vi "AI algorithm(SubVI).vi"(2 "Turn":bool, 3 "XO array":string[][](array[string])) -> (0 "Turn 2":bool, 1 "XO array 2":string[][](array[string]))   [LabVIEW 2020]
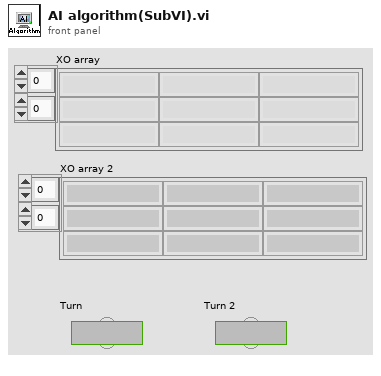
[diagram p1: front panel]
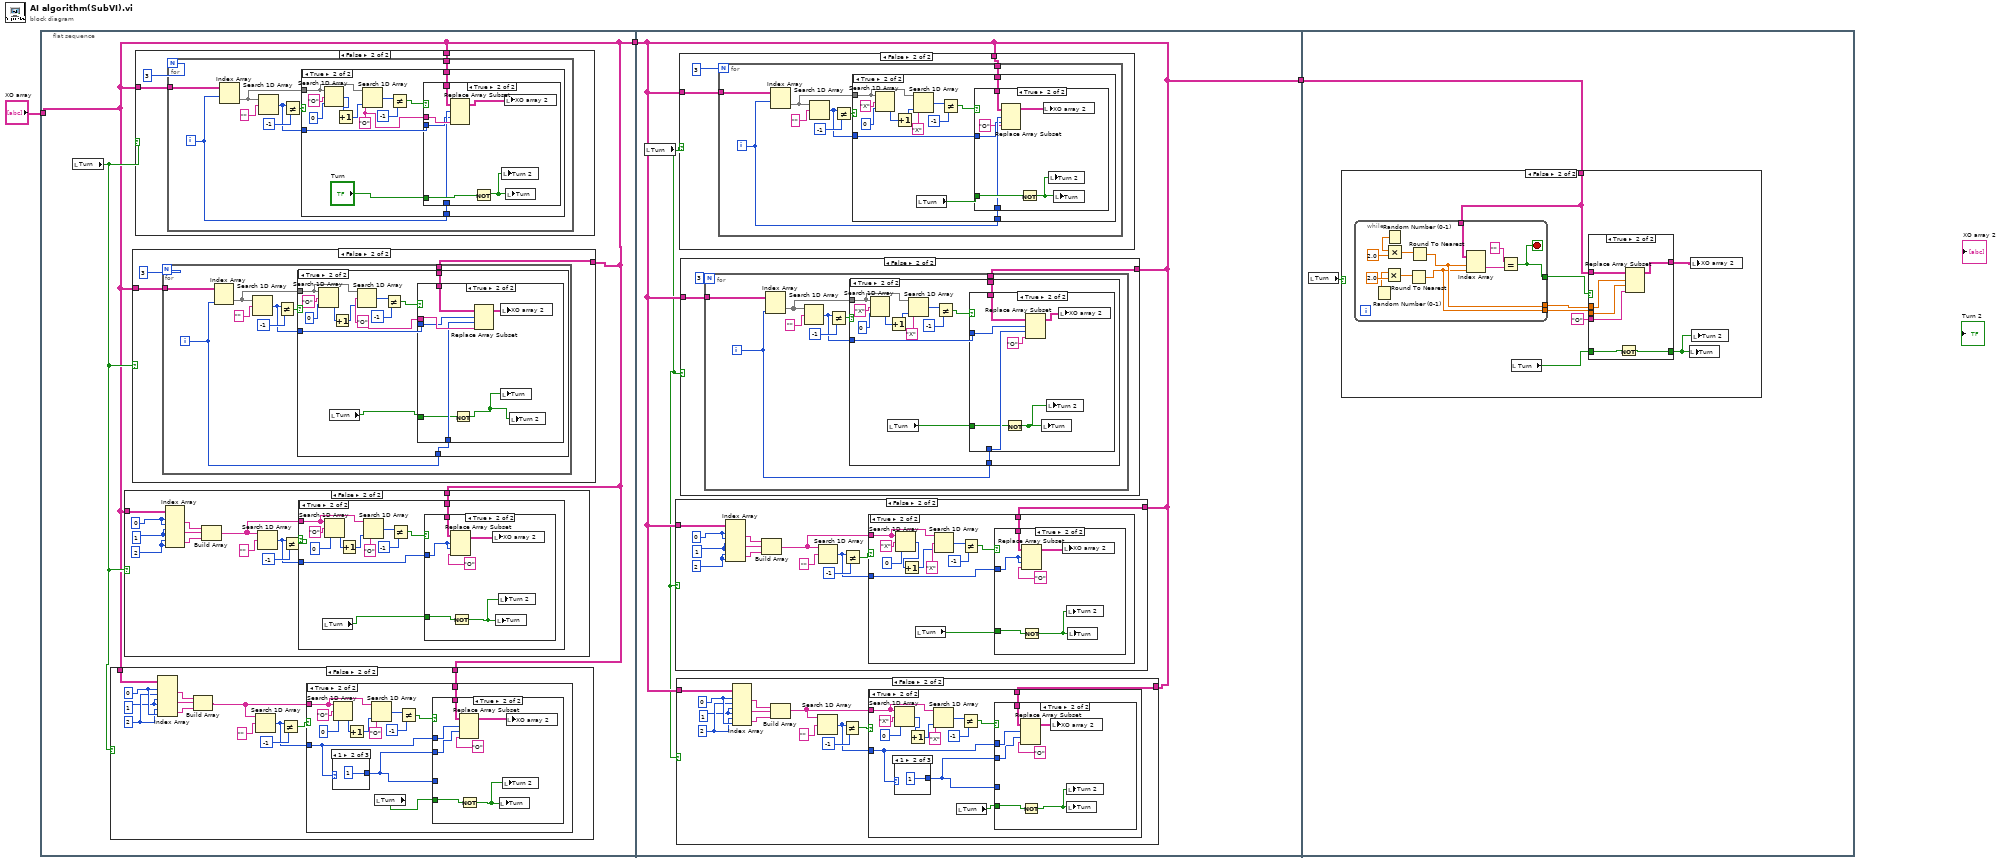
[diagram p0: block diagram]
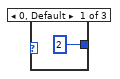
[diagram p4: hidden frame]
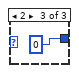
[diagram p5: hidden frame]
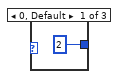
[diagram p18: hidden frame]
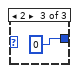
[diagram p19: hidden frame]
diagram:
  n1 = flat-sequence {
    tunnel: "XO array" -> [w4]
    tunnel: [w4] -> w2
    tunnel: w2 -> [w136]
    tunnel: [w136] -> w1
    tunnel: w1 -> [w267]
    frame #0 {
      n2 = local read "Turn"() -> (w5:bool)
      n3 = case shown="False" w5 {
        tunnel: w4 -> [_ w18]
        tunnel: w4 -> [_ w6]
        frame True {
        }
        frame False {
          w13 = 2
          w12 = 1
          w14 = 0
          n4 = Index Array(array=w18, index (row) #1=w14, index (col) #1=w13, index (row) #2=w12, index (col) #2=w12, index (row) #3=w13, index (col) #3=w14) -> (element #1=w17:string, element #2=w16:string, element #3=w15:string)
          n5 = Build Array(w17, w16, w15) -> (w7:string[])
          n6 = Search 1D Array(1D array=w7, element="") -> (index of element=w8:i32)  [unwired: 1 in]
          n7 = Not Equal?(x=w8, y=-1) -> (x != y?=w9:bool)
          n8 = case shown="True" w9 {
            tunnel: w7 -> [_ w30]
            tunnel: w8 -> [_ w24]
            tunnel: w6 -> [_ w25]
            frame False {
            }
            frame True {
              n9 = case shown="1" w24 {
                tunnel: [2 1 0] -> w23
                frame 0, Default {
                }
                frame 1 {
                }
                frame 2 {
                }
              }
              n10 = Search 1D Array(1D array=w30, element="O", start index (0)=0) -> (index of element=w22:i32)
              n11 = Increment(x=w22) -> (x+1=w21:i32)
              n12 = Search 1D Array(1D array=w30, element="O", start index (0)=w21) -> (index of element=w28:i32)
              n13 = local read "Turn"() -> (w20:bool)
              n14 = Not Equal?(x=w28, y=-1) -> (x != y?=w26:bool)
              n15 = case shown="True" w26 {
                tunnel: w24 -> [_ w39]
                tunnel: w25 -> [_ w41]
                tunnel: w20 -> [_ w38]
                tunnel: w23 -> [_ _]
                tunnel: w23 -> [_ w37]
                frame False {
                }
                frame True {
                  n16 = Replace Array Subset(array=w41, new element="O" ("new element/subarray"), index (row)=w39, index (col)=w37) -> (w36:string[][])
                  n17 = Not(x=w38) -> (.not. x?=w35:bool)
                  n18 = local write "Turn"(w35) -> ()
                  n19 = local write "Turn 2"(w35) -> ()
                  n20 = local write "XO array 2"(w36) -> ()
                }
              }
            }
          }
        }
      }
      n21 = case shown="False" w5 {
        tunnel: w4 -> [_ w54]
        tunnel: w4 -> [_ w42]
        frame True {
        }
        frame False {
          w47 = 2
          w48 = 1
          w49 = 0
          n22 = Index Array(array=w54, index (row) #1=w49, index (col) #1=w49, index (row) #2=w48, index (col) #2=w48, index (row) #3=w47, index (col) #3=w47) -> (element #1=w46:string, element #2=w45:string, element #3=w44:string)
          n23 = Build Array(w46, w45, w44) -> (w43:string[])
          n24 = Search 1D Array(1D array=w43, element="") -> (index of element=w50:i32)  [unwired: 1 in]
          n25 = Not Equal?(x=w50, y=-1) -> (x != y?=w51:bool)
          n26 = case shown="True" w51 {
            tunnel: w43 -> [_ w65]
            tunnel: w50 -> [_ w60]
            tunnel: w42 -> [_ w59]
            frame False {
            }
            frame True {
              n27 = local read "Turn"() -> (w56:bool)
              n28 = Search 1D Array(1D array=w65, element="O", start index (0)=0) -> (index of element=w58:i32)
              n29 = Increment(x=w58) -> (x+1=w57:i32)
              n30 = Search 1D Array(1D array=w65, element="O", start index (0)=w57) -> (index of element=w63:i32)
              n31 = Not Equal?(x=w63, y=-1) -> (x != y?=w61:bool)
              n32 = case shown="True" w61 {
                tunnel: w60 -> [_ w70]
                tunnel: w59 -> [_ w72]
                tunnel: w56 -> [_ w69]
                frame False {
                }
                frame True {
                  n33 = Replace Array Subset(array=w72, new element="O" ("new element/subarray"), index (row)=w70, index (col)=w70) -> (w68:string[][])
                  n34 = Not(x=w69) -> (.not. x?=w67:bool)
                  n35 = local write "XO array 2"(w68) -> ()
                  n36 = local write "Turn"(w67) -> ()
                  n37 = local write "Turn 2"(w67) -> ()
                }
              }
            }
          }
        }
      }
      n38 = case shown="False" w5 {
        tunnel: w4 -> [_ w75]
        tunnel: w4 -> [_ w73]
        frame True {
        }
        frame False {
          n39 = for {
            N: 3 -> [_]
            tunnel: w75 -> [w83]
            tunnel: w73 -> [w77]
            i -> [w76]
            n40 = Index Array(array=w83, index (col)=w76) -> (element=w79:string[])  [unwired: 1 in]
            n41 = Search 1D Array(1D array=w79, element="") -> (index of element=w78:i32)  [unwired: 1 in]
            n42 = Not Equal?(x=w78, y=-1) -> (x != y?=w80:bool)
            n43 = case shown="True" w80 {
              tunnel: w79 -> [_ w95]
              tunnel: w78 -> [_ w91]
              tunnel: w77 -> [_ w90]
              tunnel: w76 -> [_ w89]
              frame False {
              }
              frame True {
                w88 = "O" ("element")
                n44 = Search 1D Array(1D array=w95, element="O", start index (0)=0) -> (index of element=w87:i32)
                n45 = local read "Turn"() -> (w85:bool)
                n46 = Increment(x=w87) -> (x+1=w86:i32)
                n47 = Search 1D Array(1D array=w95, element=w88, start index (0)=w86) -> (index of element=w94:i32)
                n48 = Not Equal?(x=w94, y=-1) -> (x != y?=w92:bool)
                n49 = case shown="True" w92 {
                  tunnel: w91 -> [_ w100]
                  tunnel: w90 -> [_ w103]
                  tunnel: w89 -> [_ w101]
                  tunnel: w88 -> [_ w102]
                  tunnel: w85 -> [_ w99]
                  frame False {
                  }
                  frame True {
                    n50 = Not(x=w99) -> (.not. x?=w97:bool)
                    n51 = Replace Array Subset(array=w103, new element=w102, index (row)=w100, index (col)=w101) -> (w98:string[][])
                    n52 = local write "XO array 2"(w98) -> ()
                    n53 = local write "Turn"(w97) -> ()
                    n54 = local write "Turn 2"(w97) -> ()
                  }
                }
              }
            }
          }
        }
      }
      n55 = case shown="False" w5 {
        tunnel: w4 -> [_ w106]
        tunnel: w4 -> [_ w104]
        frame True {
        }
        frame False {
          n56 = for {
            N: 3 -> [_]
            tunnel: w106 -> [w114]
            tunnel: w104 -> [w108]
            i -> [w107]
            n57 = Index Array(array=w114, index (row)=w107) -> (element=w110:string[])  [unwired: 1 in]
            n58 = Search 1D Array(1D array=w110, element="") -> (index of element=w109:i32)  [unwired: 1 in]
            n59 = Not Equal?(x=w109, y=-1) -> (x != y?=w111:bool)
            n60 = case shown="True" w111 {
              tunnel: w110 -> [_ w126]
              tunnel: w109 -> [_ w122]
              tunnel: w108 -> [_ w120]
              tunnel: w107 -> [_ w119]
              frame False {
              }
              frame True {
                w121 = "O" ("element")
                n61 = Search 1D Array(1D array=w126, element="O", start index (0)=0) -> (index of element=w118:i32)
                n62 = Increment(x=w118) -> (x+1=w117:i32)
                n63 = Search 1D Array(1D array=w126, element=w121, start index (0)=w117) -> (index of element=w125:i32)
                n64 = Not Equal?(x=w125, y=-1) -> (x != y?=w123:bool)
                n65 = case shown="True" w123 {
                  tunnel: w122 -> [_ w130]
                  tunnel: w121 -> [_ w134]
                  tunnel: w120 -> [_ w133]
                  tunnel: w119 -> [_ w131]
                  tunnel: "Turn" -> [_ w132]
                  frame False {
                  }
                  frame True {
                    n66 = Replace Array Subset(array=w133, new element=w134, index (row)=w131, index (col)=w130) -> (w129:string[][])
                    n67 = Not(x=w132) -> (.not. x?=w128:bool)
                    n68 = local write "Turn 2"(w128) -> ()
                    n69 = local write "XO array 2"(w129) -> ()
                    n70 = local write "Turn"(w128) -> ()
                  }
                }
              }
            }
          }
        }
      }
    }
    frame #1 {
      n71 = local read "Turn"() -> (w135:bool)
      n72 = case shown="False" w135 {
        tunnel: w136 -> [_ w174]
        tunnel: w136 -> [_ w173]
        frame True {
        }
        frame False {
          w179 = 2
          w180 = 1
          w181 = 0
          n73 = Index Array(array=w174, index (row) #1=w181, index (col) #1=w181, index (row) #2=w180, index (col) #2=w180, index (row) #3=w179, index (col) #3=w179) -> (element #1=w178:string, element #2=w177:string, element #3=w176:string)
          n74 = Build Array(w178, w177, w176) -> (w175:string[])
          n75 = Search 1D Array(1D array=w175, element="") -> (index of element=w182:i32)  [unwired: 1 in]
          n76 = Not Equal?(x=w182, y=-1) -> (x != y?=w183:bool)
          n77 = case shown="True" w183 {
            tunnel: w175 -> [_ w196]
            tunnel: w182 -> [_ w191]
            tunnel: w173 -> [_ w190]
            frame False {
            }
            frame True {
              n78 = Search 1D Array(1D array=w196, element="X", start index (0)=0) -> (index of element=w189:i32)
              n79 = Increment(x=w189) -> (x+1=w188:i32)
              n80 = local read "Turn"() -> (w187:bool)
              n81 = Search 1D Array(1D array=w196, element="X", start index (0)=w188) -> (index of element=w194:i32)
              n82 = Not Equal?(x=w194, y=-1) -> (x != y?=w192:bool)
              n83 = case shown="True" w192 {
                tunnel: w191 -> [_ w201]
                tunnel: w190 -> [_ w203]
                tunnel: w187 -> [_ w200]
                frame False {
                }
                frame True {
                  n84 = Replace Array Subset(array=w203, new element="O" ("new element/subarray"), index (row)=w201, index (col)=w201) -> (w199:string[][])
                  n85 = Not(x=w200) -> (.not. x?=w198:bool)
                  n86 = local write "XO array 2"(w199) -> ()
                  n87 = local write "Turn 2"(w198) -> ()
                  n88 = local write "Turn"(w198) -> ()
                }
              }
            }
          }
        }
      }
      n89 = case shown="False" w135 {
        tunnel: w136 -> [_ w138]
        tunnel: w136 -> [_ w137]
        frame True {
        }
        frame False {
          w145 = 2
          w144 = 1
          w146 = 0
          n90 = Index Array(array=w137, index (row) #1=w146, index (col) #1=w145, index (row) #2=w144, index (col) #2=w144, index (row) #3=w145, index (col) #3=w146) -> (element #1=w149:string, element #2=w148:string, element #3=w147:string)
          n91 = Build Array(w149, w148, w147) -> (w139:string[])
          n92 = Search 1D Array(1D array=w139, element="") -> (index of element=w140:i32)  [unwired: 1 in]
          n93 = Not Equal?(x=w140, y=-1) -> (x != y?=w141:bool)
          n94 = case shown="True" w141 {
            tunnel: w139 -> [_ w161]
            tunnel: w140 -> [_ w155]
            tunnel: w138 -> [_ w156]
            frame False {
            }
            frame True {
              n95 = case shown="1" w155 {
                tunnel: [2 1 0] -> w154
                frame 0, Default {
                }
                frame 1 {
                }
                frame 2 {
                }
              }
              n96 = Search 1D Array(1D array=w161, element="X", start index (0)=0) -> (index of element=w153:i32)
              n97 = Increment(x=w153) -> (x+1=w152:i32)
              n98 = Search 1D Array(1D array=w161, element="X", start index (0)=w152) -> (index of element=w159:i32)
              n99 = local read "Turn"() -> (w151:bool)
              n100 = Not Equal?(x=w159, y=-1) -> (x != y?=w157:bool)
              n101 = case shown="True" w157 {
                tunnel: w155 -> [_ w170]
                tunnel: w156 -> [_ w172]
                tunnel: w151 -> [_ w169]
                tunnel: w154 -> [_ _]
                tunnel: w154 -> [_ w168]
                frame False {
                }
                frame True {
                  n102 = Replace Array Subset(array=w172, new element="O" ("new element/subarray"), index (row)=w170, index (col)=w168) -> (w167:string[][])
                  n103 = Not(x=w169) -> (.not. x?=w166:bool)
                  n104 = local write "XO array 2"(w167) -> ()
                  n105 = local write "Turn 2"(w166) -> ()
                  n106 = local write "Turn"(w166) -> ()
                }
              }
            }
          }
        }
      }
      n107 = case shown="False" w135 {
        tunnel: w136 -> [_ w237]
        tunnel: w136 -> [_ w235]
        frame True {
        }
        frame False {
          n108 = for {
            N: 3 -> [_]
            tunnel: w237 -> [w245]
            tunnel: w235 -> [w239]
            i -> [w238]
            n109 = Index Array(array=w245, index (row)=w238) -> (element=w241:string[])  [unwired: 1 in]
            n110 = Search 1D Array(1D array=w241, element="") -> (index of element=w240:i32)  [unwired: 1 in]
            n111 = Not Equal?(x=w240, y=-1) -> (x != y?=w242:bool)
            n112 = case shown="True" w242 {
              tunnel: w241 -> [_ w257]
              tunnel: w240 -> [_ w253]
              tunnel: w239 -> [_ w251]
              tunnel: w238 -> [_ w250]
              frame False {
              }
              frame True {
                n113 = Search 1D Array(1D array=w257, element="X", start index (0)=0) -> (index of element=w249:i32)
                n114 = Increment(x=w249) -> (x+1=w248:i32)
                n115 = Search 1D Array(1D array=w257, element="X", start index (0)=w248) -> (index of element=w256:i32)
                n116 = local read "Turn"() -> (w247:bool)
                n117 = Not Equal?(x=w256, y=-1) -> (x != y?=w254:bool)
                n118 = case shown="True" w254 {
                  tunnel: w253 -> [_ w262]
                  tunnel: w251 -> [_ w265]
                  tunnel: w250 -> [_ w263]
                  tunnel: w247 -> [_ w264]
                  frame False {
                  }
                  frame True {
                    n119 = Replace Array Subset(array=w265, new element="O" ("new element/subarray"), index (row)=w263, index (col)=w262) -> (w260:string[][])
                    n120 = Not(x=w264) -> (.not. x?=w259:bool)
                    n121 = local write "XO array 2"(w260) -> ()
                    n122 = local write "Turn 2"(w259) -> ()
                    n123 = local write "Turn"(w259) -> ()
                  }
                }
              }
            }
          }
        }
      }
      n124 = case shown="False" w135 {
        tunnel: w136 -> [_ w206]
        tunnel: w136 -> [_ w204]
        frame True {
        }
        frame False {
          n125 = for {
            N: 3 -> [_]
            tunnel: w206 -> [w214]
            tunnel: w204 -> [w208]
            i -> [w207]
            n126 = Index Array(array=w214, index (col)=w207) -> (element=w210:string[])  [unwired: 1 in]
            n127 = Search 1D Array(1D array=w210, element="") -> (index of element=w209:i32)  [unwired: 1 in]
            n128 = Not Equal?(x=w209, y=-1) -> (x != y?=w211:bool)
            n129 = case shown="True" w211 {
              tunnel: w210 -> [_ w226]
              tunnel: w209 -> [_ w222]
              tunnel: w208 -> [_ w221]
              tunnel: w207 -> [_ w220]
              frame False {
              }
              frame True {
                n130 = Search 1D Array(1D array=w226, element="X", start index (0)=0) -> (index of element=w218:i32)
                n131 = local read "Turn"() -> (w216:bool)
                n132 = Increment(x=w218) -> (x+1=w217:i32)
                n133 = Search 1D Array(1D array=w226, element="X", start index (0)=w217) -> (index of element=w225:i32)
                n134 = Not Equal?(x=w225, y=-1) -> (x != y?=w223:bool)
                n135 = case shown="True" w223 {
                  tunnel: w222 -> [_ w232]
                  tunnel: w221 -> [_ w234]
                  tunnel: w220 -> [_ w233]
                  tunnel: w216 -> [_ w231]
                  frame False {
                  }
                  frame True {
                    n136 = Not(x=w231) -> (.not. x?=w228:bool)
                    n137 = Replace Array Subset(array=w234, new element="O" ("new element/subarray"), index (row)=w232, index (col)=w233) -> (w229:string[][])
                    n138 = local write "Turn"(w228) -> ()
                    n139 = local write "Turn 2"(w228) -> ()
                    n140 = local write "XO array 2"(w229) -> ()
                  }
                }
              }
            }
          }
        }
      }
    }
    frame #2 {
      n141 = local read "Turn"() -> (w266:bool)
      n142 = case shown="False" w266 {
        tunnel: w267 -> [_ w270]
        frame True {
        }
        frame False {
          n143 = while {
            tunnel: [w276] -> w275
            tunnel: [w279] -> w274
            tunnel: w270 -> [w278]
            tunnel: [w277] -> w272
            stop <- w276 stop-if-true
            n144 = Random Number (0-1)() -> (number: 0 to 1=w283:dbl)
            n145 = Multiply(x=w283, y=2.0) -> (x*y=w282:dbl)
            n146 = Random Number (0-1)() -> (number: 0 to 1=w286:dbl)
            n147 = Multiply(x=w286, y=2.0) -> (x*y=w285:dbl)
            n148 = Round To Nearest(number=w282) -> (nearest integer value=w277:dbl)
            n149 = Round To Nearest(number=w285) -> (nearest integer value=w279:dbl)
            n150 = Index Array(array=w278, index (row)=w279, index (col)=w277) -> (element=w281:string)
            n151 = Equal?(x="", y=w281) -> (x = y?=w276:bool)
          }
          n152 = local read "Turn"() -> (w273:bool)
          n153 = case shown="True" w275 {
            tunnel: [w288 w296] -> w268
            tunnel: w270 -> [w289 w295]
            tunnel: w274 -> [_ w292]
            tunnel: w272 -> [_ w291]
            tunnel: "O" ("Turn") -> [_ w294]
            tunnel: [w289 w293] -> w269
            tunnel: w273 -> [w288 w290]
            frame False {
            }
            frame True {
              n154 = Not(x=w290) -> (.not. x?=w296:bool)
              n155 = Replace Array Subset(array=w295, new element=w294, index (row)=w292, index (col)=w291) -> (w293:string[][])
            }
          }
          n156 = local write "Turn"(w268) -> ()
          n157 = local write "XO array 2"(w269) -> ()
          n158 = local write "Turn 2"(w268) -> ()
        }
      }
    }
  }
